vi "Digital tube display.vi"(11 "Numeric":dbl) -> (1 "个":T1, 2 "十":T1, 3 "百":T1)   [LabVIEW 2016]
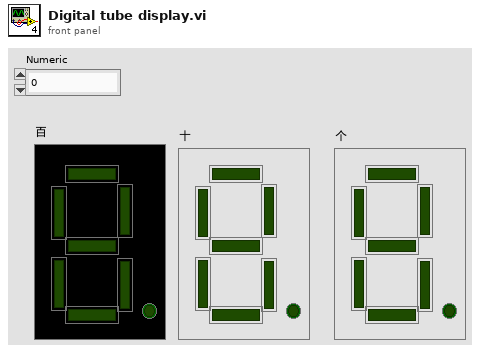
[diagram p1: front panel]
types:
  T1 = cluster{"1":bool, " 2":bool, " 3":bool, " 4":bool, " 5":bool, " 6":bool, "Boolean 7":bool, " 8":bool}
  T2 = cluster{"data[0]":bool, "data[1]":bool, "data[2]":bool, "data[3]":bool, "data[4]":bool, "data[5]":bool, "data[6]":bool, "data[7]":bool}
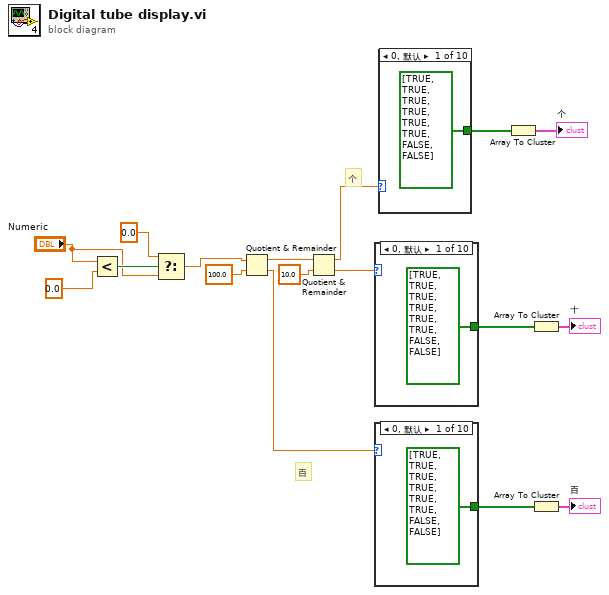
[diagram p0: block diagram]
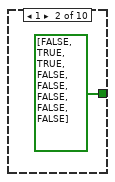
[diagram p2: hidden frame]
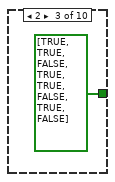
[diagram p3: hidden frame]
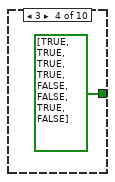
[diagram p4: hidden frame]
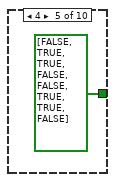
[diagram p5: hidden frame]
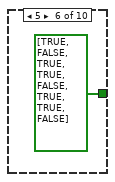
[diagram p6: hidden frame]
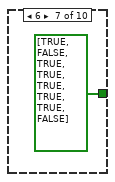
[diagram p7: hidden frame]
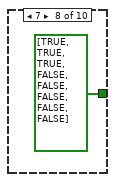
[diagram p8: hidden frame]
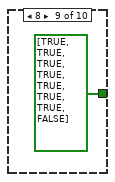
[diagram p9: hidden frame]
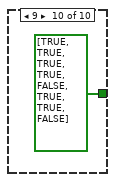
[diagram p10: hidden frame]
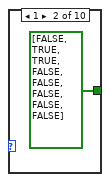
[diagram p11: hidden frame]
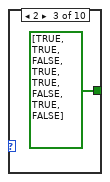
[diagram p12: hidden frame]
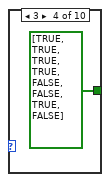
[diagram p13: hidden frame]
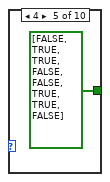
[diagram p14: hidden frame]
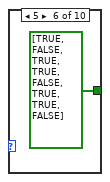
[diagram p15: hidden frame]
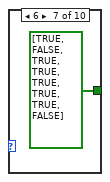
[diagram p16: hidden frame]
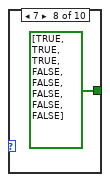
[diagram p17: hidden frame]
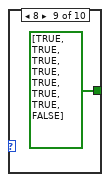
[diagram p18: hidden frame]
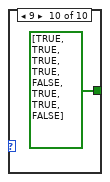
[diagram p19: hidden frame]
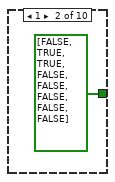
[diagram p20: hidden frame]
diagram:
  # "个"
  # "百"
  n1 = Less?(x="Numeric", y=0.0) -> (x < y?=w5:bool)
  n2 = Select(t=0.0, s=w5, f="Numeric") -> (s? t:f=w2:dbl)
  n3 = Quotient & Remainder(x=w2, y=100.0) -> (x-y*floor(x/y)=w7:dbl, floor(x/y)=w16:dbl)
  n4 = Quotient & Remainder(x=w7, y=10.0) -> (x-y*floor(x/y)=w14:dbl, floor(x/y)=w11:dbl)
  n5 = case shown="0, 默认" w11 {
    tunnel: [bool[] [TRUE, TRUE, TRUE, TRUE, TRUE, TRUE, FALSE, FALSE] ("data") bool[] [FALSE, TRUE, TRUE, FALSE, FALSE, FALSE, FALSE, FALSE] ("data") bool[] [TRUE, TRUE, FALSE, TRUE, TRUE, FALSE, TRUE, FALSE] ("data") bool[] [TRUE, TRUE, TRUE, TRUE, FALSE, FALSE, TRUE, FALSE] ("data") bool[] [FALSE, TRUE, TRUE, FALSE, FALSE, TRUE, TRUE, FALSE] ("data") bool[] [TRUE, FALSE, TRUE, TRUE, FALSE, TRUE, TRUE, FALSE] ("data") bool[] [TRUE, FALSE, TRUE, TRUE, TRUE, TRUE, TRUE, FALSE] ("data") bool[] [TRUE, TRUE, TRUE, FALSE, FALSE, FALSE, FALSE, FALSE] ("data") bool[] [TRUE, TRUE, TRUE, TRUE, TRUE, TRUE, TRUE, FALSE] ("data") bool[] [TRUE, TRUE, TRUE, TRUE, FALSE, TRUE, TRUE, FALSE] ("data")] -> w10
    frame 0, Default {
    }
    frame 1 {
    }
    frame 2 {
    }
    frame 3 {
    }
    frame 4 {
    }
    frame 5 {
    }
    frame 6 {
    }
    frame 7 {
    }
    frame 8 {
    }
    frame 9 {
    }
  }
  n6 = case shown="0, 默认" w16 {
    tunnel: [bool[] [TRUE, TRUE, TRUE, TRUE, TRUE, TRUE, FALSE, FALSE] ("data") bool[] [FALSE, TRUE, TRUE, FALSE, FALSE, FALSE, FALSE, FALSE] ("data") bool[] [TRUE, TRUE, FALSE, TRUE, TRUE, FALSE, TRUE, FALSE] ("data") bool[] [TRUE, TRUE, TRUE, TRUE, FALSE, FALSE, TRUE, FALSE] ("data") bool[] [FALSE, TRUE, TRUE, FALSE, FALSE, TRUE, TRUE, FALSE] ("data") bool[] [TRUE, FALSE, TRUE, TRUE, FALSE, TRUE, TRUE, FALSE] ("data") bool[] [TRUE, FALSE, TRUE, TRUE, TRUE, TRUE, TRUE, FALSE] ("data") bool[] [TRUE, TRUE, TRUE, FALSE, FALSE, FALSE, FALSE, FALSE] ("data") bool[] [TRUE, TRUE, TRUE, TRUE, TRUE, TRUE, TRUE, FALSE] ("data") bool[] [TRUE, TRUE, TRUE, TRUE, FALSE, TRUE, TRUE, FALSE] ("data")] -> w17
    frame 0, Default {
    }
    frame 1 {
    }
    frame 2 {
    }
    frame 3 {
    }
    frame 4 {
    }
    frame 5 {
    }
    frame 6 {
    }
    frame 7 {
    }
    frame 8 {
    }
    frame 9 {
    }
  }
  n7 = case shown="0, 默认" w14 {
    tunnel: [bool[] [TRUE, TRUE, TRUE, TRUE, TRUE, TRUE, FALSE, FALSE] ("data") bool[] [FALSE, TRUE, TRUE, FALSE, FALSE, FALSE, FALSE, FALSE] ("data") bool[] [TRUE, TRUE, FALSE, TRUE, TRUE, FALSE, TRUE, FALSE] ("data") bool[] [TRUE, TRUE, TRUE, TRUE, FALSE, FALSE, TRUE, FALSE] ("data") bool[] [FALSE, TRUE, TRUE, FALSE, FALSE, TRUE, TRUE, FALSE] ("data") bool[] [TRUE, FALSE, TRUE, TRUE, FALSE, TRUE, TRUE, FALSE] ("data") bool[] [TRUE, FALSE, TRUE, TRUE, TRUE, TRUE, TRUE, FALSE] ("data") bool[] [TRUE, TRUE, TRUE, FALSE, FALSE, FALSE, FALSE, FALSE] ("data") bool[] [TRUE, TRUE, TRUE, TRUE, TRUE, TRUE, TRUE, FALSE] ("data") bool[] [TRUE, TRUE, TRUE, TRUE, FALSE, TRUE, TRUE, FALSE] ("data")] -> w13
    frame 0, Default {
    }
    frame 1 {
    }
    frame 2 {
    }
    frame 3 {
    }
    frame 4 {
    }
    frame 5 {
    }
    frame 6 {
    }
    frame 7 {
    }
    frame 8 {
    }
    frame 9 {
    }
  }
  n8 = Array To Cluster(array=w13) -> (cluster=→"个":T2)
  n9 = Array To Cluster(array=w10) -> (cluster=→"十":T2)
  n10 = Array To Cluster(array=w17) -> (cluster=→"百":T2)
